vi "BIN_find_make_file.vi"(6 "Max Filesize (bytes)":i64 format="%.0p", 7 "Extension":string, 8 "error in":errorcluster, 9 "TAGs":string[](array[string]), 11 "OpenPattern":path) -> (0 "error out":errorcluster, 2 "New file?":bool, 3 "refnum out":refnum<file>)   [LabVIEW 2020, in "DBAL-BIN.lvclass"]
doc: "First this method will check if the week number subdirectory exists.\nIf no: then a new folder and historian file will be created with sequence number 001\nIf yes: then the weeknumber folder is searched for the latest file of this resolution layer.\nIf not found: a new file will be created with sequence number 001\nIf found: then the latest sequence of that series is searched.\nIf found and file is small enough: file is opened and reference supplied.\nIf not found or size is too large: New file with sequence number 001 is created."
uses:
  DBAL-BIN.lvclass
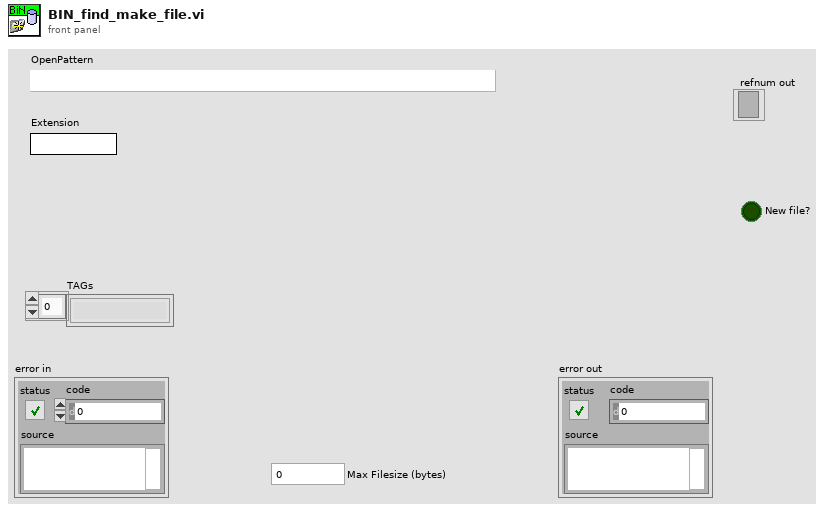
[diagram p1: front panel]
types:
  T1 = enum16{"open", "replace", "create", "open or create", "replace or create", "replace or create with confirmation"}
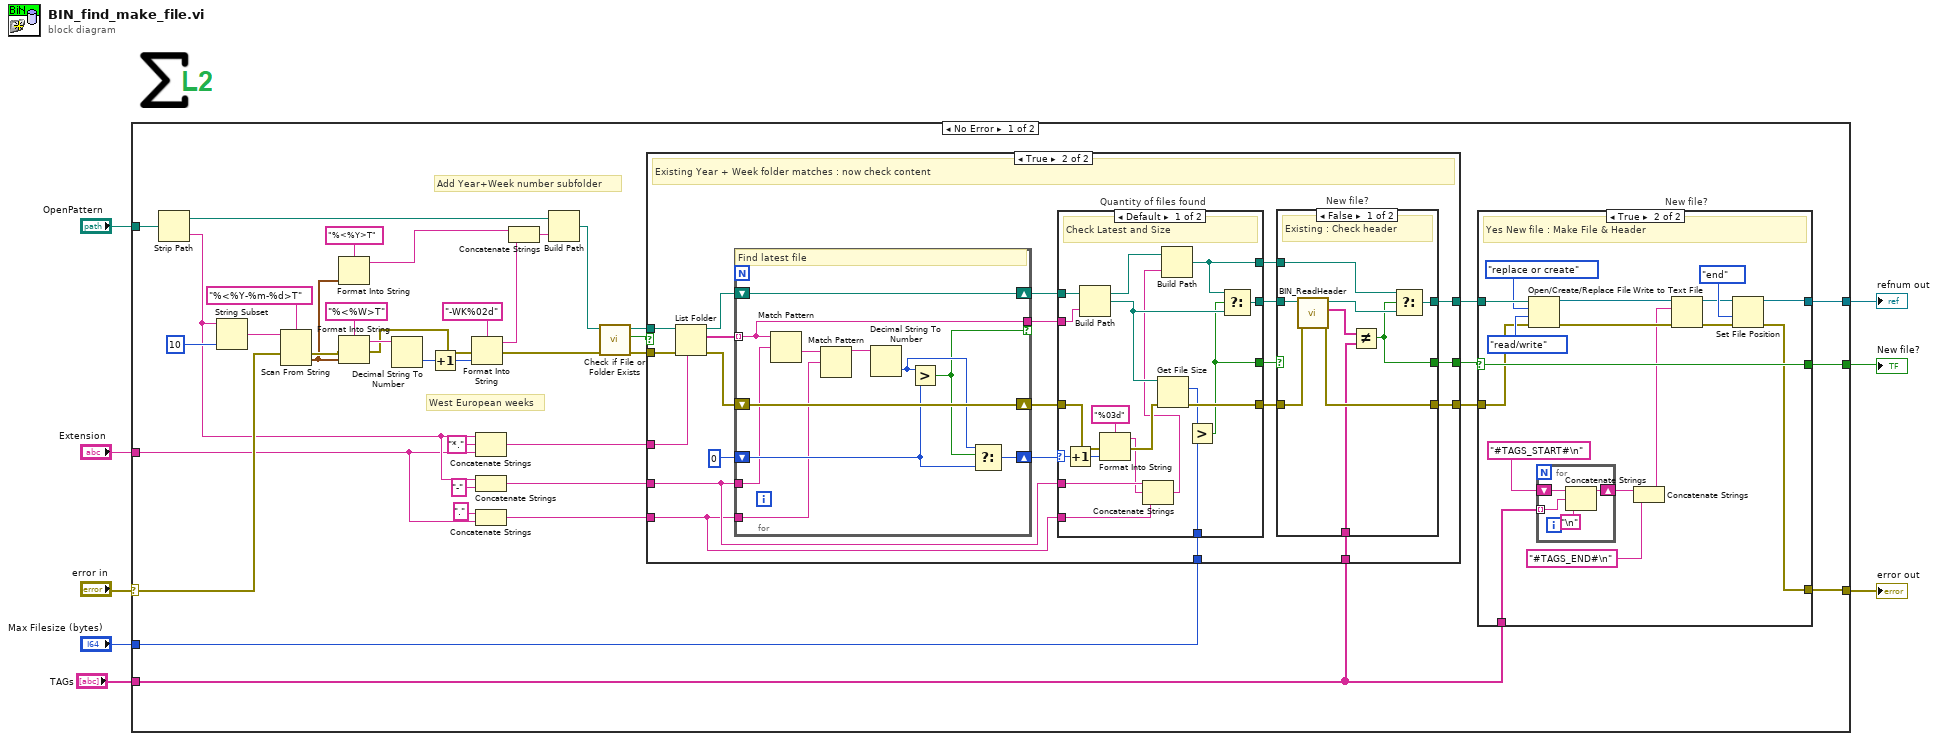
[diagram p0: block diagram]
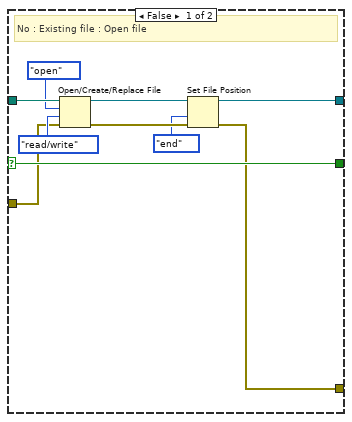
[diagram p2: hidden frame]
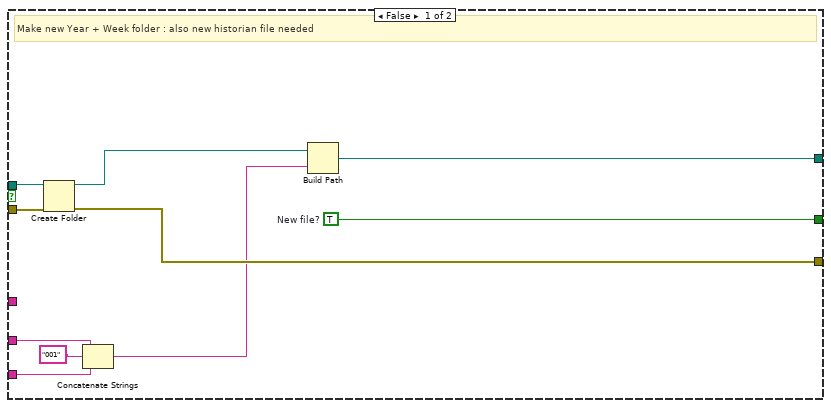
[diagram p3: hidden frame]
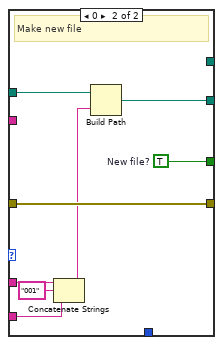
[diagram p5: hidden frame]
diagram:
  n1 = case shown="No Error" "error in" {
    selector: "error in" -> [w25 w160]
    tunnel: [w10 w160] -> w7
    tunnel: "OpenPattern" -> [w47 _]
    tunnel: "Extension" -> [w18 _]
    tunnel: "Max Filesize (bytes)" -> [w16 _]
    tunnel: "TAGs" -> [w12 _]
    tunnel: [w11 _] -> w2
    tunnel: [w9 _] -> w1
    frame No Error {
      # "West European weeks"
      # "Add Year+Week number subfolder"
      n2 = Strip Path(path=w47) -> (stripped path=w38:path, name=w22:string)
      n3 = String Subset(string=w22, length (rest)=10 ("length (rest)")) -> (substring=w45:string)  [unwired: 1 in]
      n4 = Scan From String(format string="%<%Y-%m-%d>T", input string=w45, error in=w25) -> (error out=w36:errorcluster, output 1=w32:timestamp)  [unwired: 2 in, 2 out]
      n5 = Format Into String(format string="%<%Y>T", w32) -> (resulting string=w29:string)  [unwired: 2 in, 1 out]
      n6 = Format Into String(format string="%<%W>T", error in=w36, w32) -> (resulting string=w42:string, error out=w35:errorcluster)  [unwired: 1 in]
      n7 = Decimal String To Number(string=w42) -> (number=w41:i32)  [unwired: 2 in, 1 out]
      n8 = Increment(x=w41) -> (x+1=w40:i32)
      n9 = Format Into String(format string="-WK%02d", error in=w35, w40) -> (resulting string=w31:string, error out=w34:errorcluster)  [unwired: 1 in]
      n10 = Concatenate Strings(w22, "*." ("string"), w18) -> (w23:string)
      n11 = Concatenate Strings(w22, "-" ("string")) -> (w20:string)
      n12 = Concatenate Strings("." ("string"), w18) -> (w17:string)
      n13 = Concatenate Strings(w29, w31) -> (w30:string)
      n14 = Build Path(base path=w38, name or relative path=w30) -> (appended path=w37:path)
      n15 = call <vilib>:"Check if File or Folder Exists.vi"("error in (no error)"=w34, "path"=w37) -> ("error out"=w26:errorcluster, "file or folder exists?"=w28:bool, "dup path"=w27:path)  [unwired: 7 in]
      n16 = case shown="True" w28 {
        tunnel: w27 -> [w88 w109]
        tunnel: w26 -> [w87 w110]
        tunnel: [w86 w89] -> w15
        tunnel: w23 -> [_ w108]
        tunnel: w20 -> [w81 w99]
        tunnel: w17 -> [w82 w98]
        tunnel: [w85 w90] -> w14
        tunnel: w16 -> [_ w97]
        tunnel: w12 -> [_ w93]
        tunnel: [w79 w91] -> w13
        frame False {
          w85 = TRUE  # New file?
          # "Make new Year + Week folder : also new historian file needed"
          n17 = Create Folder(path (use dialog)=w88, error in=w87) -> (created path=w84:path, error out=w86:errorcluster)  [unwired: 1 in, 1 out]
          n18 = Concatenate Strings(w81, "001" ("string"), w82) -> (w80:string)
          n19 = Build Path(base path=w84, name or relative path=w80) -> (appended path=w79:path)
        }
        frame True {
          # "Existing Year + Week folder matches : now check content"
          n20 = List Folder(path=w109, pattern=w108, error in=w110) -> (path out=w106:path, filenames=w105:string[], error out=w107:errorcluster)  [unwired: 1 in, 1 out]
          n21 = for {
            shift-right: [w157] -> w100
            shift-left: w107 -> [w157]
            shift-right: [w159] -> w102
            shift-left: w106 -> [w159]
            tunnel: w105 -> [w152] mode=indexing
            tunnel: w99 -> [w151]
            tunnel: w98 -> [w150]
            shift-right: [w153] -> w103
            shift-left: 0 -> [w154]
            tunnel: [w152] -> w101 if=w149
            # "Find latest file"
            n22 = Match Pattern(string=w152, regular expression=w151) -> (after substring=w158:string)  [unwired: 1 in, 3 out]
            n23 = Match Pattern(string=w158, regular expression=w150) -> (before substring=w156:string)  [unwired: 1 in, 3 out]
            n24 = Decimal String To Number(string=w156) -> (number=w155:i32)  [unwired: 2 in, 1 out]
            n25 = Greater?(x=w155, y=w154) -> (0:w149:bool)
            n26 = Select(t=w155, s=w149, f=w154) -> (s? t:f=w153:i32)
          }
          n27 = case "Quantity of files found" shown="Default" w103 {
            selector: w103 -> [w133 _]
            tunnel: w102 -> [w135 w147]
            tunnel: [w125 w148] -> w96
            tunnel: w101 -> [w140 _]
            tunnel: [w134 w143] -> w95
            tunnel: w99 -> [w128 w146]
            tunnel: w98 -> [w126 w144]
            tunnel: w100 -> [w130 w142]
            tunnel: [w139 w142] -> w94
            tunnel: w97 -> [w137 _]
            tunnel: [w123 _] -> w92
            frame Default {
              # "Check Latest and Size"
              n28 = Increment(x=w133) -> (x+1=w132:i32)
              n29 = Build Path(base path=w135, name or relative path=w140) -> (appended path=w136:path)
              n30 = Format Into String(format string="%03d", error in=w130, w132) -> (resulting string=w127:string, error out=w129:errorcluster)  [unwired: 1 in]
              n31 = Concatenate Strings(w128, w127, w126) -> (w124:string)
              n32 = Get File Size(file=w136, error in=w129) -> (size (in bytes)=w138:i64, 0:w139:errorcluster)  [unwired: 1 out]
              n33 = Build Path(base path=w135, name or relative path=w124) -> (appended path=w123:path)
              n34 = Greater?(x=w138, y=w137) -> (0:w125:bool)
              n35 = Select(t=w123, s=w125, f=w136) -> (s? t:f=w134:path)
            }
            frame 0 {
              w148 = TRUE  # New file?
              # "Make new file"
              n36 = Concatenate Strings(w146, "001" ("string"), w144) -> (w141:string)
              n37 = Build Path(base path=w147, name or relative path=w141) -> (appended path=w143:path)
            }
          }
          n38 = case "New file?" shown="False" w96 {
            selector: w96 -> [_ w122]
            tunnel: [w111 w122] -> w90
            tunnel: w95 -> [w117 w121]
            tunnel: [w114 w121] -> w91
            tunnel: w94 -> [w119 w120]
            tunnel: [w118 w120] -> w89
            tunnel: w93 -> [w115 _]
            tunnel: w92 -> [w112 _]
            frame False {
              # "Existing : Check header"
              n39 = call "BIN_ReadHeader.vi"("error in"=w119, "Path in"=w117) -> ("error out"=w118:errorcluster, "TAGs"=w116:string[], "Path out"=w113:path)  [unwired: 7 in]
              n40 = Not Equal?(x=w116, y=w115) -> (x != y?=w111:bool)
              n41 = Select(t=w112, s=w111, f=w113) -> (s? t:f=w114:path)
            }
            frame True {
              # "New : no action here"
            }
          }
        }
      }
      n42 = case "New file?" shown="True" w14 {
        selector: w14 -> [w57 w74]
        tunnel: [w57 w74] -> w11
        tunnel: w13 -> [w56 w73]
        tunnel: [w52 w58] -> w9
        tunnel: w15 -> [w50 w70]
        tunnel: [w49 w61] -> w10
        tunnel: w12 -> [_ w69]
        frame False {
          # "No : Existing file : Open file"
          n43 = Open/Create/Replace File(file path (use dialog)=w56, error in=w50, operation (0:open)=T1."open", access (0:read/write)=enum16{"read/write", "read-only", "write-only"}."read/write") -> (refnum out=w53:refnum<file>, error out=w51:errorcluster)  [unwired: 2 in, 1 out]
          n44 = Set File Position(refnum=w53, from (0:start)=enum16{"start", "end", "current"}."end", error in=w51) -> (refnum out=w52:refnum<file>, error out=w49:errorcluster)  [unwired: 1 in]
        }
        frame True {
          # "Yes New file : Make File & Header"
          n45 = Open/Create/Replace File(file path (use dialog)=w73, error in=w70, operation (0:open)=T1."replace or create", access (0:read/write)=enum16{"read/write", "read-only", "write-only"}."read/write") -> (refnum out=w64:refnum<file>, error out=w62:errorcluster)  [unwired: 2 in, 1 out]
          n46 = for {
            tunnel: w69 -> [w77] mode=indexing
            shift-right: [w76] -> w67
            shift-left: "#TAGS_START#\n" -> [w78]
            n47 = Concatenate Strings(w78, w77, "\n") -> (w76:string)
          }
          n48 = Concatenate Strings(w67, "#TAGS_END#\n") -> (w60:string)
          n49 = Write to Text File(file (use dialog)=w64, text=w60, error in=w62) -> (refnum out=w59:refnum<file>, error out=w63:errorcluster)  [unwired: 1 in, 1 out]
          n50 = Set File Position(refnum=w59, from (0:start)=enum16{"start", "end", "current"}."end", error in=w63) -> (refnum out=w58:refnum<file>, error out=w61:errorcluster)  [unwired: 1 in]
        }
      }
    }
    frame Error {
    }
  }
  "error out" <- w7
  "New file?" <- w2
  "refnum out" <- w1
